vi "Type Info.vi"(11 "Build Package Item in":refnum<class "VIPM Item.lvclass">) -> (1 "Description":string, 2 "Pretty Name":string, 3 "Type":string)   [LabVIEW 2019, in "VIPM.lvlib" / "VIPM Item.lvclass"]
doc: "Returns Type information about the solution item.\n----\nCopyright: MGI 2017\nAuthor: Derek Trepanier"
uses:
  VIPM Item.lvclass
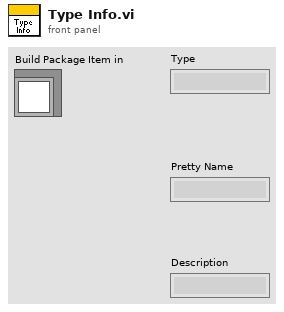
[diagram p1: front panel]
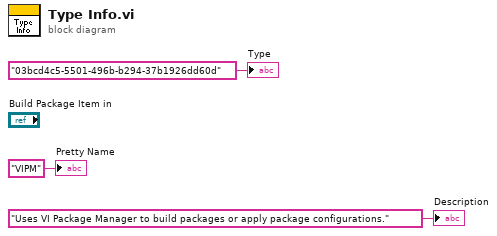
[diagram p0: block diagram]
diagram:
  "Pretty Name" <- "VIPM" ("Pretty Name")
  "Description" <- "Uses VI Package Manager to build packages or apply package configurations." ("Description")
  "Type" <- "03bcd4c5-5501-496b-b294-37b1926dd60d" ("Type")
